vi "Create_New_Array_for_Comparason.vi"(1 "Captured Plots":T1(array[cluster])) -> (0 "Generated Distance Array":dbl[][](array[numeric]))   [LabVIEW 2012]
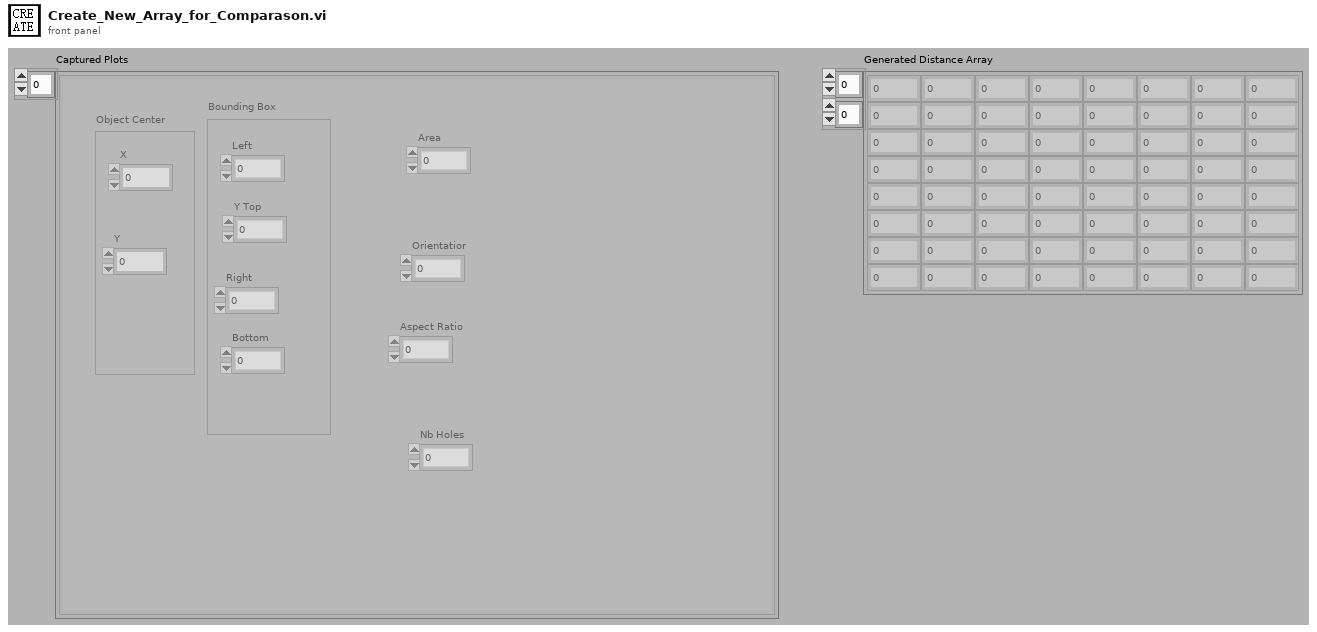
[diagram p1: front panel]
types:
  T1 = cluster{"Object Center":cluster{"X":dbl, "Y":dbl}, "Bounding Box":cluster{"Left":dbl, "Right":dbl, "Bottom":dbl, "Y Top":dbl}, "Area":dbl, "Orientatior":dbl, "Aspect Ratio":dbl, "Nb Holes":dbl}[]
  T2 = cluster{"Object Center":cluster{"X":dbl, "Y":dbl}, "Bounding Box":cluster{"Left":dbl, "Right":dbl, "Bottom":dbl, "Y Top":dbl}, "Area":dbl, "Orientatior":dbl, "Aspect Ratio":dbl, "Nb Holes":dbl}
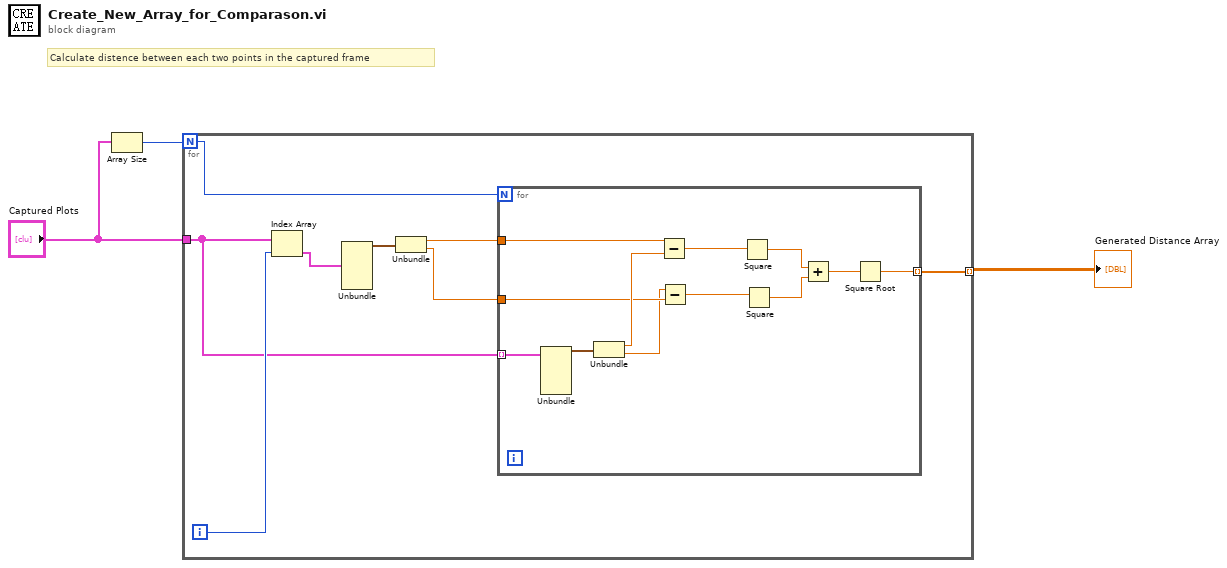
[diagram p0: block diagram]
diagram:
  # "Calculate distence between each two points in the captured frame"
  n1 = Array Size(array="Captured Plots") -> (size(s)=w3:i32)
  n2 = for {
    N: w3 -> [w4]
    tunnel: "Captured Plots" -> [w10]
    tunnel: [w8] -> w1 mode=indexing
    i -> [w11]
    n3 = Index Array(array=w10, index=w11) -> (element=w9:T2)
    n4 = Unbundle(w9) -> ("Object Center"=w7:cluster{"X":dbl, "Y":dbl})  [unwired: 5 out]
    n5 = Unbundle(w7) -> ("X"=w6:dbl, "Y"=w5:dbl)
    n6 = for {
      N: w4 -> [_]
      tunnel: w10 -> [w23] mode=indexing
      tunnel: [w18] -> w8 mode=indexing
      tunnel: w6 -> [w14]
      tunnel: w5 -> [w13]
      n7 = Unbundle(w23) -> ("Object Center"=w16:cluster{"X":dbl, "Y":dbl})  [unwired: 5 out]
      n8 = Unbundle(w16) -> ("X"=w15:dbl, "Y"=w12:dbl)
      n9 = Subtract(x=w14, y=w15) -> (x-y=w22:dbl)
      n10 = Subtract(x=w12, y=w13) -> (x-y=w21:dbl)
      n11 = Square(x=w22) -> (x^2=w20:dbl)
      n12 = Square(x=w21) -> (x^2=w19:dbl)
      n13 = Add(x=w20, y=w19) -> (x+y=w17:dbl)
      n14 = Square Root(x=w17) -> (sqrt(x)=w18:dbl)
    }
  }
  "Generated Distance Array" <- w1
